vi "Get update instructions.vi"(8 "error in (no error)":errorcluster, 10 "only position":bool, 11 "Motor in":refnum<class "Motor.lvclass">) -> (0 "error out":errorcluster, 1 "name":string, 2 "read instructions":string[](array[string]), 3 "Motor out":refnum<class "Motor.lvclass">)   [LabVIEW 2018, in "Motor.lvclass"]
uses:
  Motor.lvclass
  Motor.lvclass/Motor.ctl
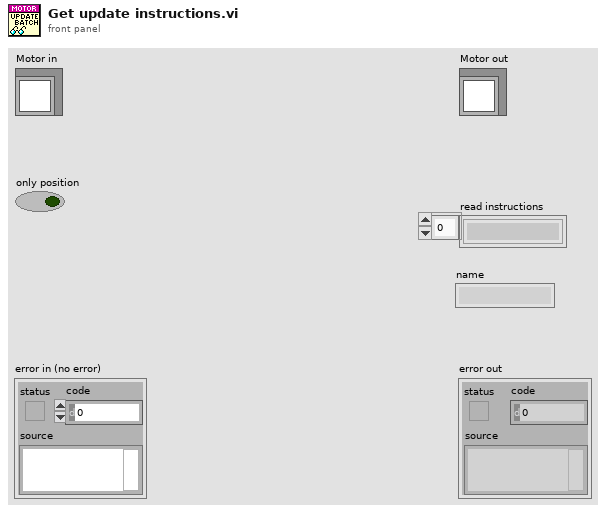
[diagram p1: front panel]
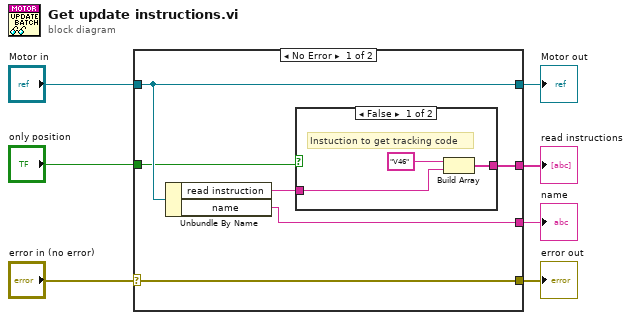
[diagram p0: block diagram]
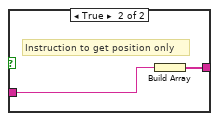
[diagram p2: hidden frame]
diagram:
  n1 = case shown="No Error" "error in (no error)" {
    selector: "error in (no error)" -> [w13 w19]
    tunnel: [w13 w19] -> w6
    tunnel: [w11 w20] -> w4
    tunnel: "Motor in" -> [w11 w20]
    tunnel: [w12 _] -> w3
    tunnel: "only position" -> [w10 _]
    tunnel: [w8 _] -> w1
    frame No Error {
      n2 = Unbundle By Name(w11) -> ("read instruction"=w9:string, "name"=w8:string)
      n3 = case shown="False" w10 {
        tunnel: [w15 w17] -> w12
        tunnel: w9 -> [w14 w18]
        frame False {
          # "Instuction to get tracking code"
          n4 = Build Array("V46", w14) -> (w15:string[])
        }
        frame True {
          # "Instruction to get position only"
          n5 = Build Array(w18) -> (w17:string[])
        }
      }
    }
    frame Error {
    }
  }
  "error out" <- w6
  "Motor out" <- w4
  "read instructions" <- w3
  "name" <- w1
